vi "setOutputState.vi"(8 "error in (no error)":errorcluster, 10 "Output State":bool, 11 "FgenNiPxi in":refnum<class "ArbNi.lvclass">) -> (0 "error out":errorcluster, 3 "FgenNiPxi out":refnum<class "ArbNi.lvclass">)   [LabVIEW 2023, in "ArbNi.lvclass"]
doc: "<b>Author:</b> Wolfgang\n<b>Description:</b> Set Output Voltage Amplitude Vpk"
uses:
  ArbNi.lvclass
  ArbNi.lvclass/ArbNi.ctl
  Arb.lvclass
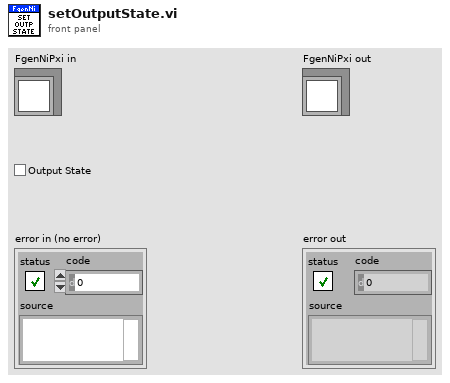
[diagram p1: front panel]
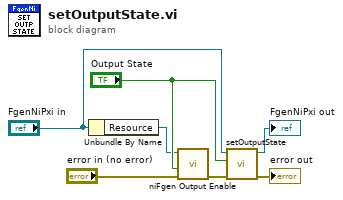
[diagram p0: block diagram]
diagram:
  n1 = Unbundle By Name("FgenNiPxi in") -> ("Resource"=w1:refnum<k15>)
  n2 = call <instrlib>:"niFgen Output Enable.vi"("error in (no error)"="error in (no error)", "Output Enable (default: True)"="Output State", "Instrument Handle"=w1) -> ("error out"=w3:errorcluster)  [unwired: 7 in, 1 out]
  n3 = call-parent "setOutputState.vi"("error in (no error)"=w3, "Output State"="Output State", "Fgen in"="FgenNiPxi in") -> ("error out"=→"error out":errorcluster, "Fgen out"=→"FgenNiPxi out":refnum<class "ArbNi.lvclass">)  [unwired: 7 in]
